vi "Setscale.vi"(8 "error in (no error)":errorcluster, 10 "Array":T1(array[cluster]), 11 "WaveformChart in":T2) -> (0 "error out":errorcluster, 2 "Value":T1(array[cluster]), 3 "WaveformChart out":T2)   [LabVIEW 2016]
uses:
  Typedefs/HitChart refnum.ctl
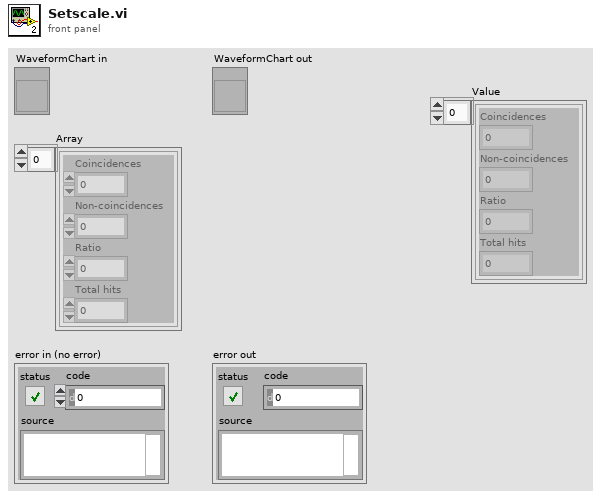
[diagram p1: front panel]
types:
  T1 = cluster{"Coincidences":dbl, "Non-coincidences":dbl, "Ratio":dbl, "Total hits":dbl}[]
  T2 = typedef "HitChart refnum.ctl" = refnum<vi>
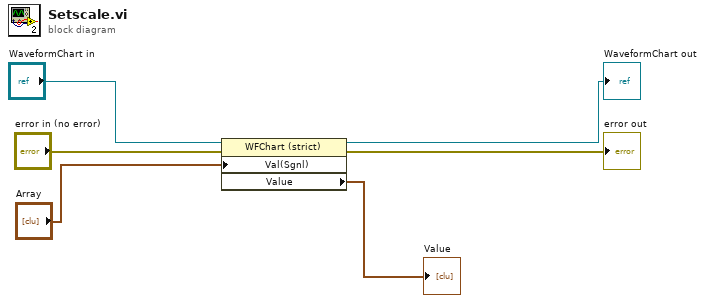
[diagram p0: block diagram]
diagram:
  n1 = property class="WFChart (strict)"(reference="WaveformChart in", error in="error in (no error)", "Val(Sgnl)"="Array") -> (reference out=→"WaveformChart out":T2, error out=→"error out":errorcluster, "Value"=→"Value":T1)
